vi "Select axis.vi"(0 "System No.":i32=1 min=1 max=4 step=1, 2 "Axes in":string[](array[string])) -> (14 "Selected axis":string, 15 "Index of axis\nin Global 2":i32, 16 "Index of axis\nin Axes in array":i32)   [LabVIEW 2020]
doc: "This VI reads all connected axes from Global2 and writes them into a menu ring control for selection. The selected axis and its index in Global2 are returned."
panel:
  in  "Available\naxes":u16(ring) items=["X", "Y", "Z", "U", "V", "W"]
  in  "Select":bool
  # "Select axis"
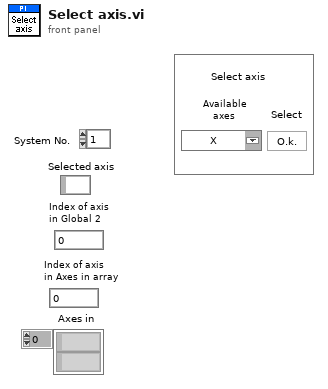
[diagram p1: front panel]
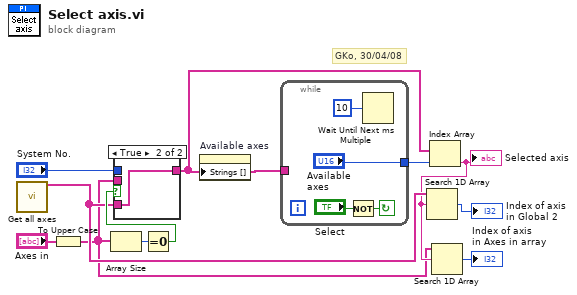
[diagram p0: block diagram]
diagram:
  # "GKo, 30/04/08"
  n1 = call "Get all axes.vi"() -> ("Conn. Axes"=w4:string[])  [unwired: 1 in, 18 out]
  n2 = To Upper Case(1:"Axes in") -> (0:w1:string[])
  n3 = Array Size(array=w1) -> (size(s)=w8:i32)
  n4 = Equal To 0?(x=w8) -> (x = 0?=w7:bool)
  n5 = case shown="True" w7 {
    tunnel: [w12 w13] -> w10
    tunnel: "System No." -> [_ _]
    tunnel: w1 -> [w12 _]
    tunnel: w4 -> [_ w13]
    frame False {
    }
    frame True {
    }
  }
  n6 = property on="Available axes" class="Ring (strict)"("Strings []"=w10) -> ()  [unwired: 2 in, 2 out]
  n7 = while {
    tunnel: ["Available\naxes"] -> w11
    tunnel: w10 -> [_]
    stop <- w16 continue-if-true
    n8 = Not(x="Select") -> (.not. x?=w16:bool)
    n9 = Wait Until Next ms Multiple(millisecond multiple=u32 10) -> ()  [unwired: 1 out]
  }
  n10 = Index Array(array=w10, index=w11) -> (element=w2:string)
  "Selected axis" <- w2
  n11 = Search 1D Array(1D array=w4, element=w2) -> (index of element=→"Index of axis\nin Global 2":i32)  [unwired: 1 out]
  n12 = Search 1D Array(1D array=w1, element=w2) -> (index of element=→"Index of axis\nin Axes in array":i32)  [unwired: 1 out]
